vi "ParseObj.vi"(4 "String":string) -> (0 "BuildingInfoArray":T1(array[cluster]), 1 "FaceArray":T3(array[cluster]) {"zNorm" format="%.2f"; "yNorm" format="%.2f"; "xNorm" format="%.2f"; "zVert" format="%^#_6g"; "yVert" format="%^#_6g"; "xVert" format="%^#_6g"}, 2 "SiteAverage":cluster{"x":dbl, "y":dbl, "z":dbl})   [LabVIEW 2010]
panel:
  out "lastLoop":bool
  out "BuildMin":cluster{"x":dbl, "y":dbl, "z":dbl}
  out "BuildMax":cluster{"x":dbl, "y":dbl, "z":dbl}
  out "BuildingInfo":T2
  out "BldgStartVertex":u32
  out "BuildAverage":cluster{"x":dbl, "y":dbl, "z":dbl}
  out "VertexCount":u32
  out "FaceCount":u32
  out "Array":string[][](array[string])
  out "offset past match":i32
  out "Loop":i32
  out "StringPosition":i32
  out "BuildingCount":u32
  out "CurrentBuildingName":string
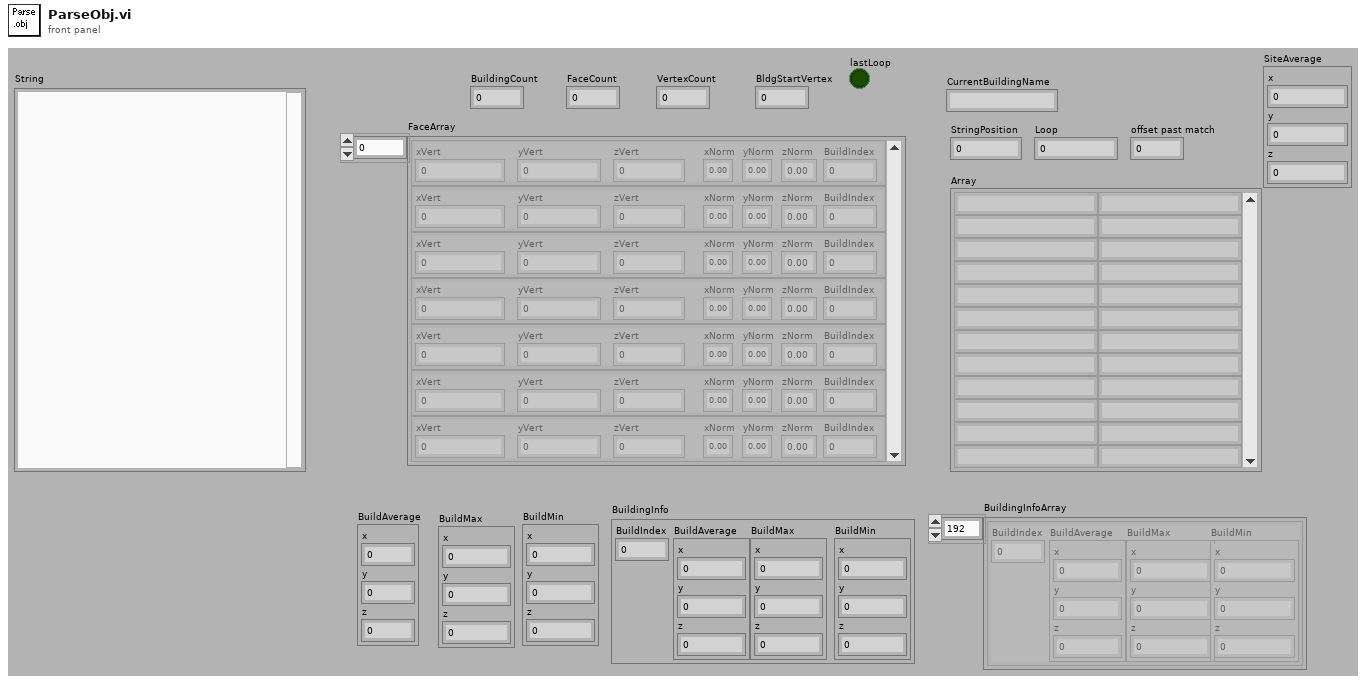
[diagram p1: front panel]
types:
  T1 = cluster{"BuildAverage":cluster{"x":dbl, "y":dbl, "z":dbl}, "BuildIndex":u32, "BuildMax":cluster{"x":dbl, "y":dbl, "z":dbl}, "BuildMin":cluster{"x":dbl, "y":dbl, "z":dbl}}[]
  T2 = cluster{"BuildAverage":cluster{"x":dbl, "y":dbl, "z":dbl}, "BuildIndex":u32, "BuildMax":cluster{"x":dbl, "y":dbl, "z":dbl}, "BuildMin":cluster{"x":dbl, "y":dbl, "z":dbl}}
  T3 = cluster{"xVert":dbl, "yVert":dbl, "zVert":dbl, "xNorm":dbl, "yNorm":dbl, "zNorm":dbl, "BuildIndex":u32}[]
  T4 = cluster{"xVert":dbl, "yVert":dbl, "zVert":dbl, "xNorm":dbl, "yNorm":dbl, "zNorm":dbl, "BuildIndex":u32}
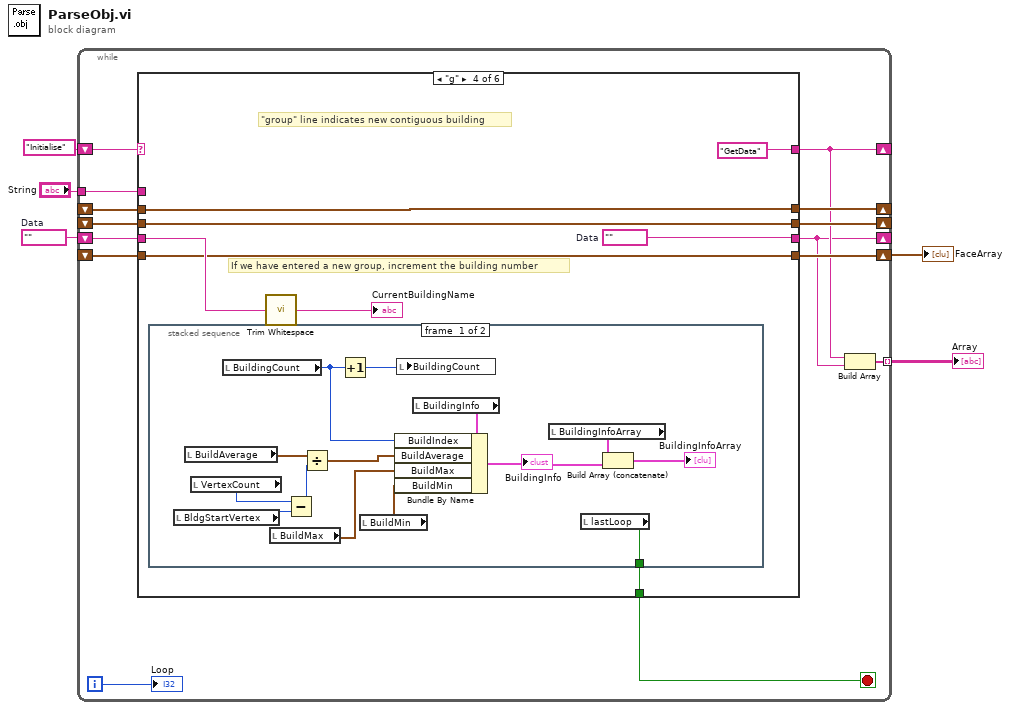
[diagram p0: block diagram]
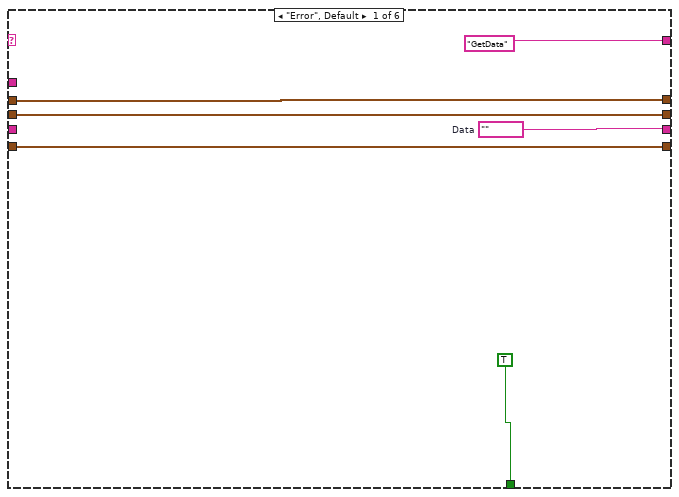
[diagram p2: hidden frame]
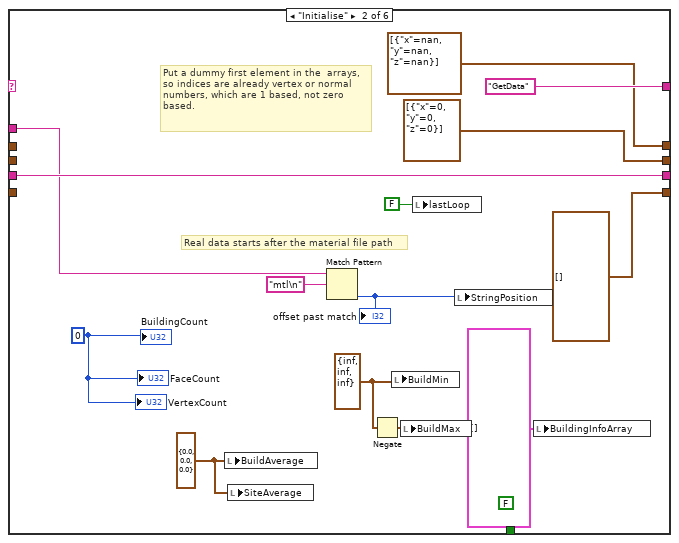
[diagram p3: hidden frame]
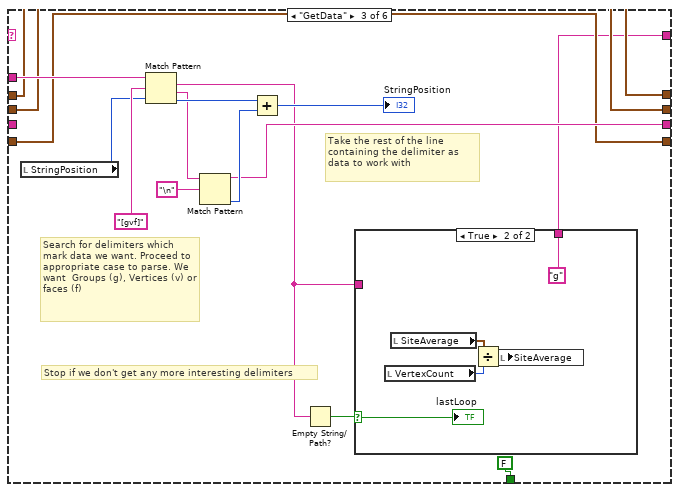
[diagram p4: hidden frame]
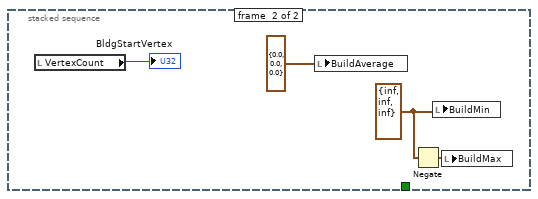
[diagram p6: hidden frame]
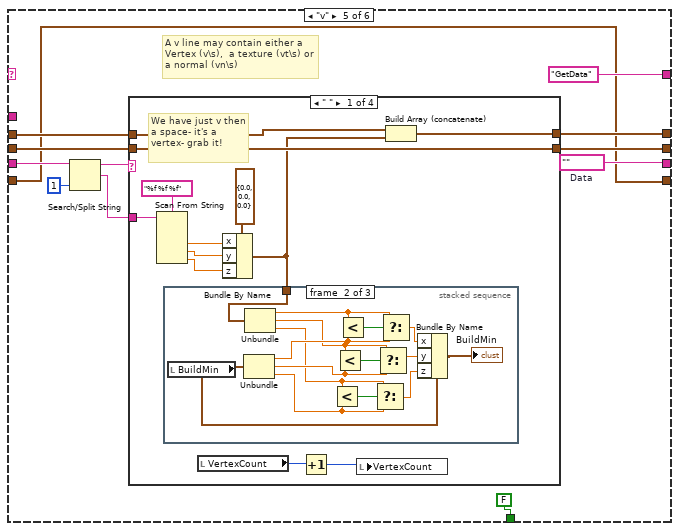
[diagram p7: hidden frame]
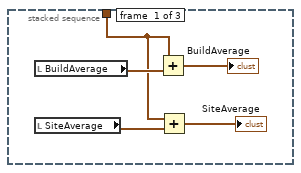
[diagram p8: hidden frame]
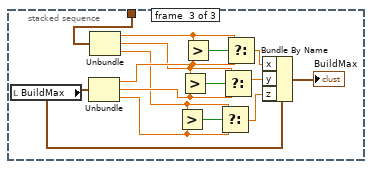
[diagram p9: hidden frame]
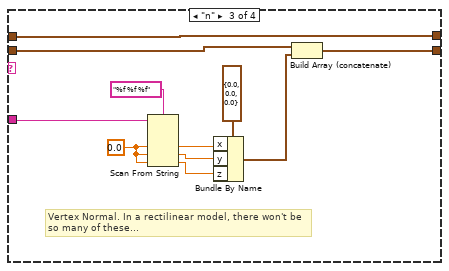
[diagram p11: hidden frame]
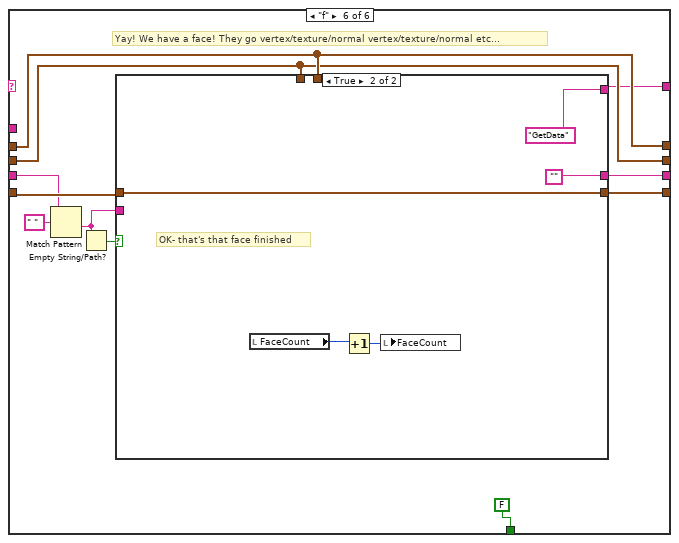
[diagram p13: hidden frame]
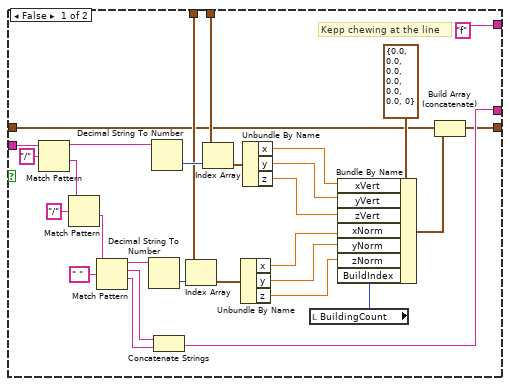
[diagram p14: hidden frame]
diagram:
  w3 = ""  # Data
  n1 = while {
    tunnel: "String" -> [w19]
    shift-right: [w8] -> _
    shift-left: "Initialise" -> [w17]
    shift-right: [w7] -> _
    shift-left: w3 -> [w16]
    shift-right: [w14] -> _
    shift-left: _ -> [w15]
    shift-right: [w13] -> _
    shift-left: _ -> [w12]
    shift-right: [w11] -> w2
    shift-left: _ -> [w10]
    tunnel: [w6] -> w1 mode=indexing
    i -> [w9]
    stop <- w18 stop-if-true
    n2 = case shown="\"g\"" w17 {
      tunnel: w19 -> [_ w34 w55 _ _ _]
      tunnel: [TRUE FALSE FALSE w63 FALSE FALSE] -> w18
      tunnel: ["GetData" "GetData" ("String") w42 "GetData" "GetData" w168] -> w8
      tunnel: [w23 w39 w50 w69 w99 w167] -> w7
      tunnel: w16 -> [_ w39 _ w68 w97 w164]
      tunnel: w15 -> [w22 _ w48 w66 w93 w171]
      tunnel: [w22 cluster{"x":dbl, "y":dbl, "z":dbl}[] [{"x"=nan, "y"=nan, "z"=nan}] ("VertexArray") w48 w66 w92 w171] -> w14
      tunnel: [w21 cluster{"x":i8, "y":i8, "z":i8}[] [{"x"=0, "y"=0, "z"=0}] ("NormalArray") w47 w65 w91 w170] -> w13
      tunnel: w12 -> [w21 _ w47 w65 w90 w170]
      tunnel: [w20 T3 [] w46 w64 w89 w166] -> w11
      tunnel: w10 -> [w20 _ w46 w64 w89 w165]
      frame "Error", Default {
        w23 = ""  # Data
      }
      frame "Initialise" {
        w28 = cluster{"x":dbl, "y":dbl, "z":dbl} {"x"=inf, "y"=inf, "z"=inf} ("BuildMin")
        w27 = cluster{"x":dbl, "y":dbl, "z":dbl} {"x"=0.0, "y"=0.0, "z"=0.0} ("Building Average")
        w32 = u32 0 ("BuildingIndex")
        # "Put a dummy first element in the  arrays, so indices are already vertex or normal numbers, which are 1 based, not zero based."
        # "Real data starts after the material file path"
        n3 = local write "BuildAverage"(w27) -> ()
        n4 = local write "SiteAverage"(w27) -> ()
        n5 = Match Pattern(string=w34, regular expression="mtl\n") -> (offset past match=w33:i32)  [unwired: 4 out]
        "offset past match" <- w33
        n6 = Negate(x=w28) -> (-x=w29:cluster{"x":dbl, "y":dbl, "z":dbl})
        n7 = local write "BuildMin"(w28) -> ()
        n8 = local write "BuildMax"(w29) -> ()
        n9 = local write "lastLoop"(FALSE ("lastLoop")) -> ()
        n10 = local write "StringPosition"(w33) -> ()
        n11 = local write "BuildingInfoArray"(T1 [] ("BuildingInfoArray")) -> ()
        "FaceCount" <- w32
        "VertexCount" <- w32
        "BuildingCount" <- w32
      }
      frame "GetData" {
        # "Stop if we don't get any more interesting delimiters"
        # "Take the rest of the line containing the delimiter as data to work with"
        # "Search for delimiters which mark data we want. Proceed to appropriate case to parse. We want  Groups (g), Vertices (v) or faces (f)"
        n12 = local read "StringPosition"() -> (w49:i32)
        n13 = Match Pattern(string=w55, regular expression="[gvf]", offset (0)=w49) -> (match substring=w43:string, after substring=w53:string, offset past match=w54:i32)  [unwired: 1 out]
        n14 = Match Pattern(string=w53, regular expression="\n") -> (before substring=w50:string, offset past match=w51:i32)  [unwired: 3 out]
        n15 = Add(x=w54, y=w51) -> (x+y=→"StringPosition":i32)
        n16 = Empty String/Path?(string/path=w43) -> (empty?=w44:bool)
        n17 = case shown="True" w44 {
          selector: w44 -> [_ w59]
          tunnel: [w57 "g" ("String")] -> w42
          tunnel: w43 -> [w57 _]
          frame False {
          }
          frame True {
            n18 = local read "VertexCount"() -> (w61:u32)
            n19 = local read "SiteAverage"() -> (w62:cluster{"x":dbl, "y":dbl, "z":dbl})
            n20 = Divide(x=w62, y=w61) -> (x/y=w60:cluster{"x":dbl, "y":dbl, "z":dbl})
            n21 = local write "SiteAverage"(w60) -> ()
            "lastLoop" <- w59
          }
        }
      }
      frame "g" {
        w69 = ""  # Data
        # "If we have entered a new group, increment the building number"
        # "\"group\" line indicates new contiguous building"
        n22 = stacked-sequence {
          tunnel: [w71 _] -> w63
          frame #0 {
            n23 = local read "BldgStartVertex"() -> (w74:u32)
            n24 = local read "BuildAverage"() -> (w81:cluster{"x":dbl, "y":dbl, "z":dbl})
            n25 = local read "VertexCount"() -> (w75:u32)
            n26 = local read "BuildingCount"() -> (w82:u32)
            n27 = local read "BuildMax"() -> (w77:cluster{"x":dbl, "y":dbl, "z":dbl})
            n28 = Subtract(x=w75, y=w74) -> (x-y=w73:u32)
            n29 = Divide(x=w81, y=w73) -> (x/y=w76:cluster{"x":dbl, "y":dbl, "z":dbl})
            n30 = Increment(x=w82) -> (x+1=w84:u32)
            n31 = local read "BuildMin"() -> (w72:cluster{"x":dbl, "y":dbl, "z":dbl})
            n32 = local write "BuildingCount"(w84) -> ()
            n33 = local read "BuildingInfo"() -> (w83:T2)
            n34 = Bundle By Name(cluster=w83, "BuildIndex"=w82, "BuildAverage"=w76, "BuildMax"=w77, "BuildMin"=w72) -> (w78:T2)
            "BuildingInfo" <- w78
            n35 = local read "BuildingInfoArray"() -> (w79:T1)
            n36 = local read "lastLoop"() -> (w71:bool)
            n37 = Build Array (concatenate)(w79, w78) -> (→"BuildingInfoArray":T1)
          }
          frame #1 {
            w85 = cluster{"x":dbl, "y":dbl, "z":dbl} {"x"=inf, "y"=inf, "z"=inf} ("BuildMin")
            n38 = local read "VertexCount"() -> (→"BldgStartVertex":u32)
            n39 = local write "BuildAverage"(cluster{"x":dbl, "y":dbl, "z":dbl} {"x"=0.0, "y"=0.0, "z"=0.0} ("Building Average")) -> ()
            n40 = Negate(x=w85) -> (-x=w86:cluster{"x":dbl, "y":dbl, "z":dbl})
            n41 = local write "BuildMin"(w85) -> ()
            n42 = local write "BuildMax"(w86) -> ()
          }
        }
        n43 = call <vilib>:"Trim Whitespace.vi"("string"=w68) -> ("trimmed string"=→"CurrentBuildingName":string)  [unwired: 1 in]
      }
      frame "v" {
        w99 = ""  # Data
        # "A v line may contain either a Vertex (v\\s),  a texture (vt\\s) or a normal (vn\\s)"
        n44 = Search/Split String(string=w97, offset (0)=1) -> (substring before match=w95:string, match + rest of string=w94:string)  [unwired: 2 out]
        n45 = case shown="\" \"" w95 {
          tunnel: w94 -> [w112 _ w154 _]
          tunnel: w93 -> [w108 w149 w160 w162]
          tunnel: [w107 w149 w160 w162] -> w92
          tunnel: [w104 w148 w151 w161] -> w91
          tunnel: w90 -> [w104 w148 w153 w161]
          frame " " {
            # "We have just v then a space- it's a vertex- grab it!"
            n46 = Scan From String(format string="%f %f %f", input string=w112) -> (output 1=w111:dbl, output 2=w110:dbl, output 3=w109:dbl)  [unwired: 2 in, 6 out]
            n47 = local read "VertexCount"() -> (w103:u32)
            n48 = Bundle By Name(cluster=cluster{"x":dbl, "y":dbl, "z":dbl} {"x"=0.0, "y"=0.0, "z"=0.0} ("VertexClusterTemplate"), "x"=w111, "y"=w110, "z"=w109) -> (w102:cluster{"x":dbl, "y":dbl, "z":dbl})
            n49 = stacked-sequence {
              tunnel: w102 -> [w115 w129 w145]
              frame #0 {
                n50 = local read "BuildAverage"() -> (w116:cluster{"x":dbl, "y":dbl, "z":dbl})
                n51 = local read "SiteAverage"() -> (w114:cluster{"x":dbl, "y":dbl, "z":dbl})
                n52 = Add(x=w115, y=w116) -> (x+y=→"BuildAverage":cluster{"x":dbl, "y":dbl, "z":dbl})
                n53 = Add(x=w115, y=w114) -> (x+y=→"SiteAverage":cluster{"x":dbl, "y":dbl, "z":dbl})
              }
              frame #1 {
                n54 = local read "BuildMin"() -> (w128:cluster{"x":dbl, "y":dbl, "z":dbl})
                n55 = Unbundle(w128) -> ("x"=w126:dbl, "y"=w122:dbl, "z"=w121:dbl)
                n56 = Unbundle(w129) -> ("x"=w127:dbl, "y"=w123:dbl, "z"=w120:dbl)
                n57 = Less?(x=w120, y=w121) -> (x < y?=w124:bool)
                n58 = Less?(x=w123, y=w122) -> (x < y?=w125:bool)
                n59 = Less?(x=w127, y=w126) -> (x < y?=w130:bool)
                n60 = Select(t=w120, s=w124, f=w121) -> (s? t:f=w118:dbl)
                n61 = Select(t=w123, s=w125, f=w122) -> (s? t:f=w119:dbl)
                n62 = Select(t=w127, s=w130, f=w126) -> (s? t:f=w131:dbl)
                n63 = Bundle By Name(cluster=w128, "x"=w131, "y"=w119, "z"=w118) -> (→"BuildMin":cluster{"x":dbl, "y":dbl, "z":dbl})
              }
              frame #2 {
                n64 = local read "BuildMax"() -> (w144:cluster{"x":dbl, "y":dbl, "z":dbl})
                n65 = Unbundle(w144) -> ("x"=w142:dbl, "y"=w138:dbl, "z"=w137:dbl)
                n66 = Unbundle(w145) -> ("x"=w143:dbl, "y"=w139:dbl, "z"=w136:dbl)
                n67 = Greater?(x=w136, y=w137) -> (0:w140:bool)
                n68 = Greater?(x=w139, y=w138) -> (0:w141:bool)
                n69 = Greater?(x=w143, y=w142) -> (0:w146:bool)
                n70 = Select(t=w136, s=w140, f=w137) -> (s? t:f=w134:dbl)
                n71 = Select(t=w139, s=w141, f=w138) -> (s? t:f=w135:dbl)
                n72 = Select(t=w143, s=w146, f=w142) -> (s? t:f=w147:dbl)
                n73 = Bundle By Name(cluster=w144, "x"=w147, "y"=w135, "z"=w134) -> (→"BuildMax":cluster{"x":dbl, "y":dbl, "z":dbl})
              }
            }
            n74 = Increment(x=w103) -> (x+1=w101:u32)
            n75 = local write "VertexCount"(w101) -> ()
            n76 = Build Array (concatenate)(w108, w102) -> (w107:cluster{"x":dbl, "y":dbl, "z":dbl}[])
          }
          frame "t" {
            # "Ignore vertex texture descriptions"
          }
          frame "n" {
            w150 = 0.0 ("default value 1")
            # "Vertex Normal. In a rectilinear model, there won't be so many of these..."
            n77 = Scan From String(format string="%f %f %f", input string=w154, default 1=w150, default 2=w150, default 3=w150) -> (output 1=w159:dbl, output 2=w158:dbl, output 3=w157:dbl)  [unwired: 2 in, 3 out]
            n78 = Bundle By Name(cluster=cluster{"x":dbl, "y":dbl, "z":dbl} {"x"=0.0, "y"=0.0, "z"=0.0} ("NormalClusterTemplate"), "x"=w159, "y"=w158, "z"=w157) -> (w152:cluster{"x":dbl, "y":dbl, "z":dbl})
            n79 = Build Array (concatenate)(w153, w152) -> (w151:cluster{"x":dbl, "y":dbl, "z":dbl}[])
          }
          frame "Error", Default {
            # "v was followed by something different! Should never happen..."
          }
        }
      }
      frame "f" {
        # "Yay! We have a face! They go vertex/texture/normal vertex/texture/normal etc..."
        n80 = Match Pattern(string=w164, regular expression=" ") -> (after substring=w163:string)  [unwired: 4 out]
        n81 = Empty String/Path?(string/path=w163) -> (empty?=w169:bool)
        n82 = case shown="True" w169 {
          tunnel: w171 -> [w197 _]
          tunnel: w170 -> [w188 _]
          tunnel: ["f" "GetData"] -> w168
          tunnel: [w180 ""] -> w167
          tunnel: [w177 w206] -> w166
          tunnel: w165 -> [w175 w206]
          tunnel: w163 -> [w174 _]
          frame False {
            # "Kepp chewing at the line"
            n83 = Match Pattern(string=w174, regular expression="/") -> (before substring=w199:string, after substring=w191:string)  [unwired: 3 out]
            n84 = Match Pattern(string=w191, regular expression="/") -> (after substring=w190:string)  [unwired: 4 out]
            n85 = Match Pattern(string=w190, regular expression=" ") -> (before substring=w183:string, match substring=w179:string, after substring=w181:string)  [unwired: 2 out]
            n86 = Decimal String To Number(string=w183) -> (number=w189:i32)  [unwired: 3 out]
            n87 = Decimal String To Number(string=w199) -> (number=w198:i32)  [unwired: 3 out]
            n88 = Concatenate Strings(w179, w181) -> (w180:string)
            n89 = Index Array(array=w188, index=w189) -> (element=w187:cluster{"x":dbl, "y":dbl, "z":dbl})
            n90 = Index Array(array=w197, index=w198) -> (element=w196:cluster{"x":dbl, "y":dbl, "z":dbl})
            n91 = Unbundle By Name(w187) -> ("x"=w186:dbl, "y"=w185:dbl, "z"=w184:dbl)
            n92 = Unbundle By Name(w196) -> ("x"=w195:dbl, "y"=w194:dbl, "z"=w193:dbl)
            n93 = local read "BuildingCount"() -> (w201:u32)
            n94 = Bundle By Name(cluster=T4 {"xVert"=0.0, "yVert"=0.0, "zVert"=0.0, "xNorm"=0.0, "yNorm"=0.0, "zNorm"=0.0, "BuildIndex"=0} ("FaceClusterTemplate"), "xVert"=w195, "yVert"=w194, "zVert"=w193, "xNorm"=w186, "yNorm"=w185, "zNorm"=w184, "BuildIndex"=w201) -> (w176:T4)
            n95 = Build Array (concatenate)(w175, w176) -> (w177:T3)
          }
          frame True {
            # "OK- that's that face finished"
            n96 = local read "FaceCount"() -> (w204:u32)
            n97 = Increment(x=w204) -> (x+1=w203:u32)
            n98 = local write "FaceCount"(w203) -> ()
          }
        }
      }
    }
    n99 = Build Array(w8, w7) -> (w6:string[])
    "Loop" <- w9
  }
  "FaceArray" <- w2
  "Array" <- w1
